vi "Find First Tag Header.vi"(8 "Error In":errorcluster, 11 "XML String":string) -> (0 "Error Out":errorcluster, 3 "After First Tag String":string, 4 "Parsing Info":T2, 5 "Parsed Header":T1)   [LabVIEW 2020, in "NI_VIAnCFGDataStructure.lvlib" / "Tree.lvclass"]
uses:
  <vilib>/addons/analyzer/VIAnCFGDataStructure/Tree Manager/Tree.lvclass
  <vilib>/addons/analyzer/VIAnCFGDataStructure/Tree Manager/Private/Parsing Info.ctl
  <vilib>/addons/analyzer/VIAnCFGDataStructure/Tree Manager/Private/Parsed Header.ctl
  <vilib>/dlg_ctls.llb/Space Constant.vi
  <vilib>/Utility/error.llb/Error Cluster From Error Code.vi
  <vilib>/addons/analyzer/VIAnCFGDataStructure/Tree Manager/API/Split String Tree.vi
  <vilib>/Utility/error.llb/Trim Whitespace.vi
  <vilib>/ErrorRing/Error Ring.xnode
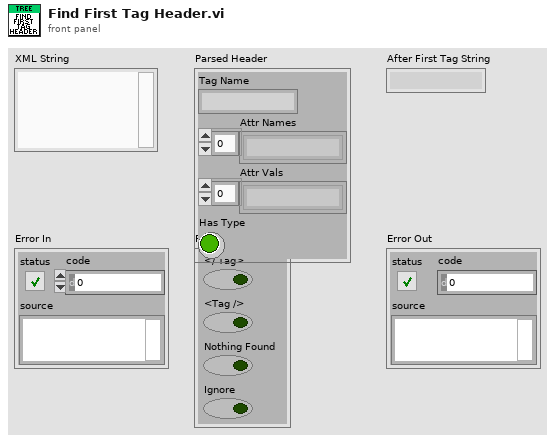
[diagram p1: front panel]
types:
  T1 = typedef "NI_VIAnCFGDataStructure.lvlib/Tree.lvclass/Parsed Header.ctl" = cluster{"Tag Name":string, "Attr Names":string[], "Attr Vals":string[], "Has Type":bool}
  T2 = typedef "NI_VIAnCFGDataStructure.lvlib/Tree.lvclass/Parsing Info.ctl" = cluster{"</ Tag>":bool, "<Tag />":bool, "Nothing Found":bool, "Ignore":bool}
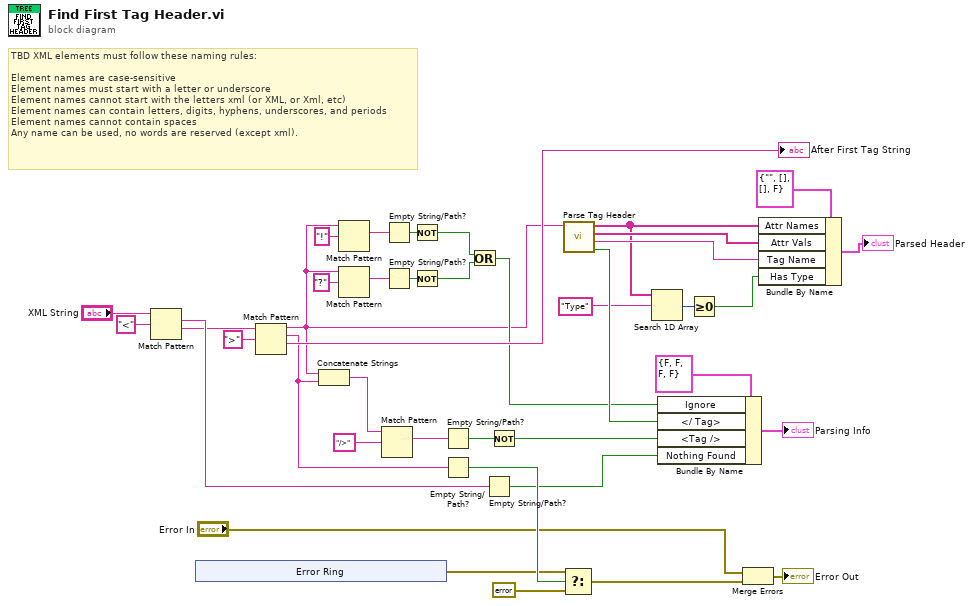
[diagram p0: block diagram]
diagram:
  # "TBD XML elements must follow these naming rules:\n\nElement names are case-sensitive\nElement names must start with a letter or underscore\nElement names cannot start with the letters xml (or XML, or Xml, etc)\nElement names can contain letters, digits, hyphens, underscores, and periods\nElement names cannot contain spaces\nAny name can be used, no words are reserved (except xml)."
  n1 = Match Pattern(string="XML String", regular expression="<") -> (match substring=w37:string, after substring=w9:string)  [unwired: 1 in, 2 out]
  n2 = xnode "Error Ring"() -> ("error out"=w26:errorcluster)
  n3 = Match Pattern(string=w9, regular expression=">") -> (before substring=w5:string, match substring=w29:string, after substring=→"After First Tag String":string)  [unwired: 1 in, 1 out]
  n4 = Concatenate Strings(w5, w29) -> (w28:string)
  n5 = Match Pattern(string=w5, regular expression="!") -> (match substring=w11:string)  [unwired: 1 in, 3 out]
  n6 = Match Pattern(string=w5, regular expression="?") -> (match substring=w14:string)  [unwired: 1 in, 3 out]
  n7 = Match Pattern(string=w28, regular expression="/>") -> (match substring=w35:string)  [unwired: 1 in, 3 out]
  n8 = Empty String/Path?(string/path=w11) -> (empty?=w12:bool)
  n9 = Empty String/Path?(string/path=w14) -> (empty?=w13:bool)
  n10 = Not(x=w12) -> (.not. x?=w7:bool)
  n11 = Not(x=w13) -> (.not. x?=w8:bool)
  n12 = Empty String/Path?(string/path=w35) -> (empty?=w32:bool)
  n13 = Empty String/Path?(string/path=w29) -> (empty?=w27:bool)
  n14 = Or(x=w7, y=w8) -> (x .or. y?=w6:bool)
  n15 = Empty String/Path?(string/path=w37) -> (empty?=w24:bool)
  n16 = Not(x=w32) -> (.not. x?=w25:bool)
  n17 = Select(t=w26, s=w27, f=errorcluster {"status"=FALSE, "code"=0, "source"=""}) -> (s? t:f=w19:errorcluster)
  n18 = call <vilib>:"Parse Tag Header.vi"("Tag Header String"=w5) -> ("</ Tag>"=w33:bool, "Tag Name"=w20:string, "Attr Vals"=w22:string[], "Attr Names"=w2:string[])  [unwired: 7 in]
  n19 = Search 1D Array(1D array=w2, element="Type") -> (index of element=w3:i32)  [unwired: 1 in]
  n20 = Bundle By Name(cluster=T2 {"</ Tag>"=FALSE, "<Tag />"=FALSE, "Nothing Found"=FALSE, "Ignore"=FALSE}, "Ignore"=w6, "</ Tag>"=w33, "<Tag />"=w25, "Nothing Found"=w24) -> (→"Parsing Info":T2)
  n21 = Greater Or Equal To 0?(x=w3) -> (x >= 0?=w1:bool)
  n22 = Merge Errors("Error In", w19) -> (→"Error Out":errorcluster)
  n23 = Bundle By Name(cluster=T1 {"Tag Name"="", "Attr Names"=[], "Attr Vals"=[], "Has Type"=FALSE} ("output cluster"), "Attr Names"=w2, "Attr Vals"=w22, "Tag Name"=w20, "Has Type"=w1) -> (→"Parsed Header":T1)
